vi "Main_TwoLoopsV3.vi"() -> ()   [LabVIEW 2022 SP3]
uses:
  SubVIs/ENUMs/StateENUM.ctl
  <vilib>/Instr/_visa.llb/VISA Configure Serial Port (Instr).vi
  <vilib>/ptbypt/NI_PtbyPt.lvlib
panel:
  in  "Enable PID":bool
  in  "Delay (sec)":dbl=5.0
  in  "Target Pressure":dbl=50.0
  out "Systole":dbl
  out "Diastole":dbl
  out "MAP":dbl
  out "Waveform Chart":dbl(graph)
  in  "Check Center":bool
  out "Step":i32
  in  "Increase Step":bool
  in  "Decrease Step":bool
  out "Center":i32
  out "LoopCount":i32
  in  "Jitter Up":bool
  in  "Jitter Down":bool
  out "Command Buffer":string
  in  "stop":bool
  out "Current Time":timestamp format="%<%I:%M:%S %p | %m/%d/%y>T"
  in  "VISA resource name":refnum<visa-resource-name>="COM9"
  in  "Up Button":bool
  in  "Down Button":bool
  # "Manual\nAdjustment"
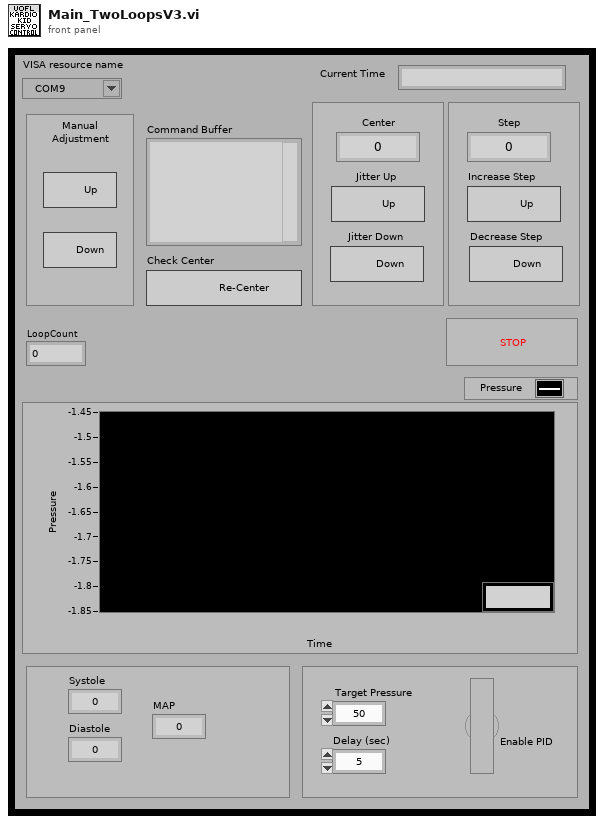
[diagram p1: front panel]
types:
  T1 = typedef "StateENUM.ctl" = enum16{"Init", "Idle", "MoveUp", "MoveDown", "JitterUp", "JitterDown", "IncreaseStep", "DecreaseStep", "CheckCenter", "ReadSerial", "ScanData", "Shutdown"}
  T2 = cluster{"Time Stamp":timestamp, "Delay":dbl, "PIDEnabled?":bool, "Target Pressure":dbl, "MAP":dbl}
  T3 = cluster{"State":T1, "Stop":bool, "error out":errorcluster}
  T4 = typedef "MoveCommands.ctl" = cluster{"MoveUp":string, "MoveDown":string, "JitterUp":string, "JitterDown":string, "IncStep":string, "DecStep":string, "ChkCenter":string}
  T5 = cluster{"VISA resource name out":refnum<visa-resource-name>, "error out":errorcluster, "State":T1, "Stop":bool, "Buffer":string, "Center":i32, "Step":i32, "SerialIncoming?":bool, "MoveCommands":T4}
  T6 = cluster{"Command Buffer":refnum<vi>, "Jitter Up":refnum<vi>, "Jitter Down":refnum<vi>, "Increase Step":refnum<vi>, "Decrease Step":refnum<vi>}
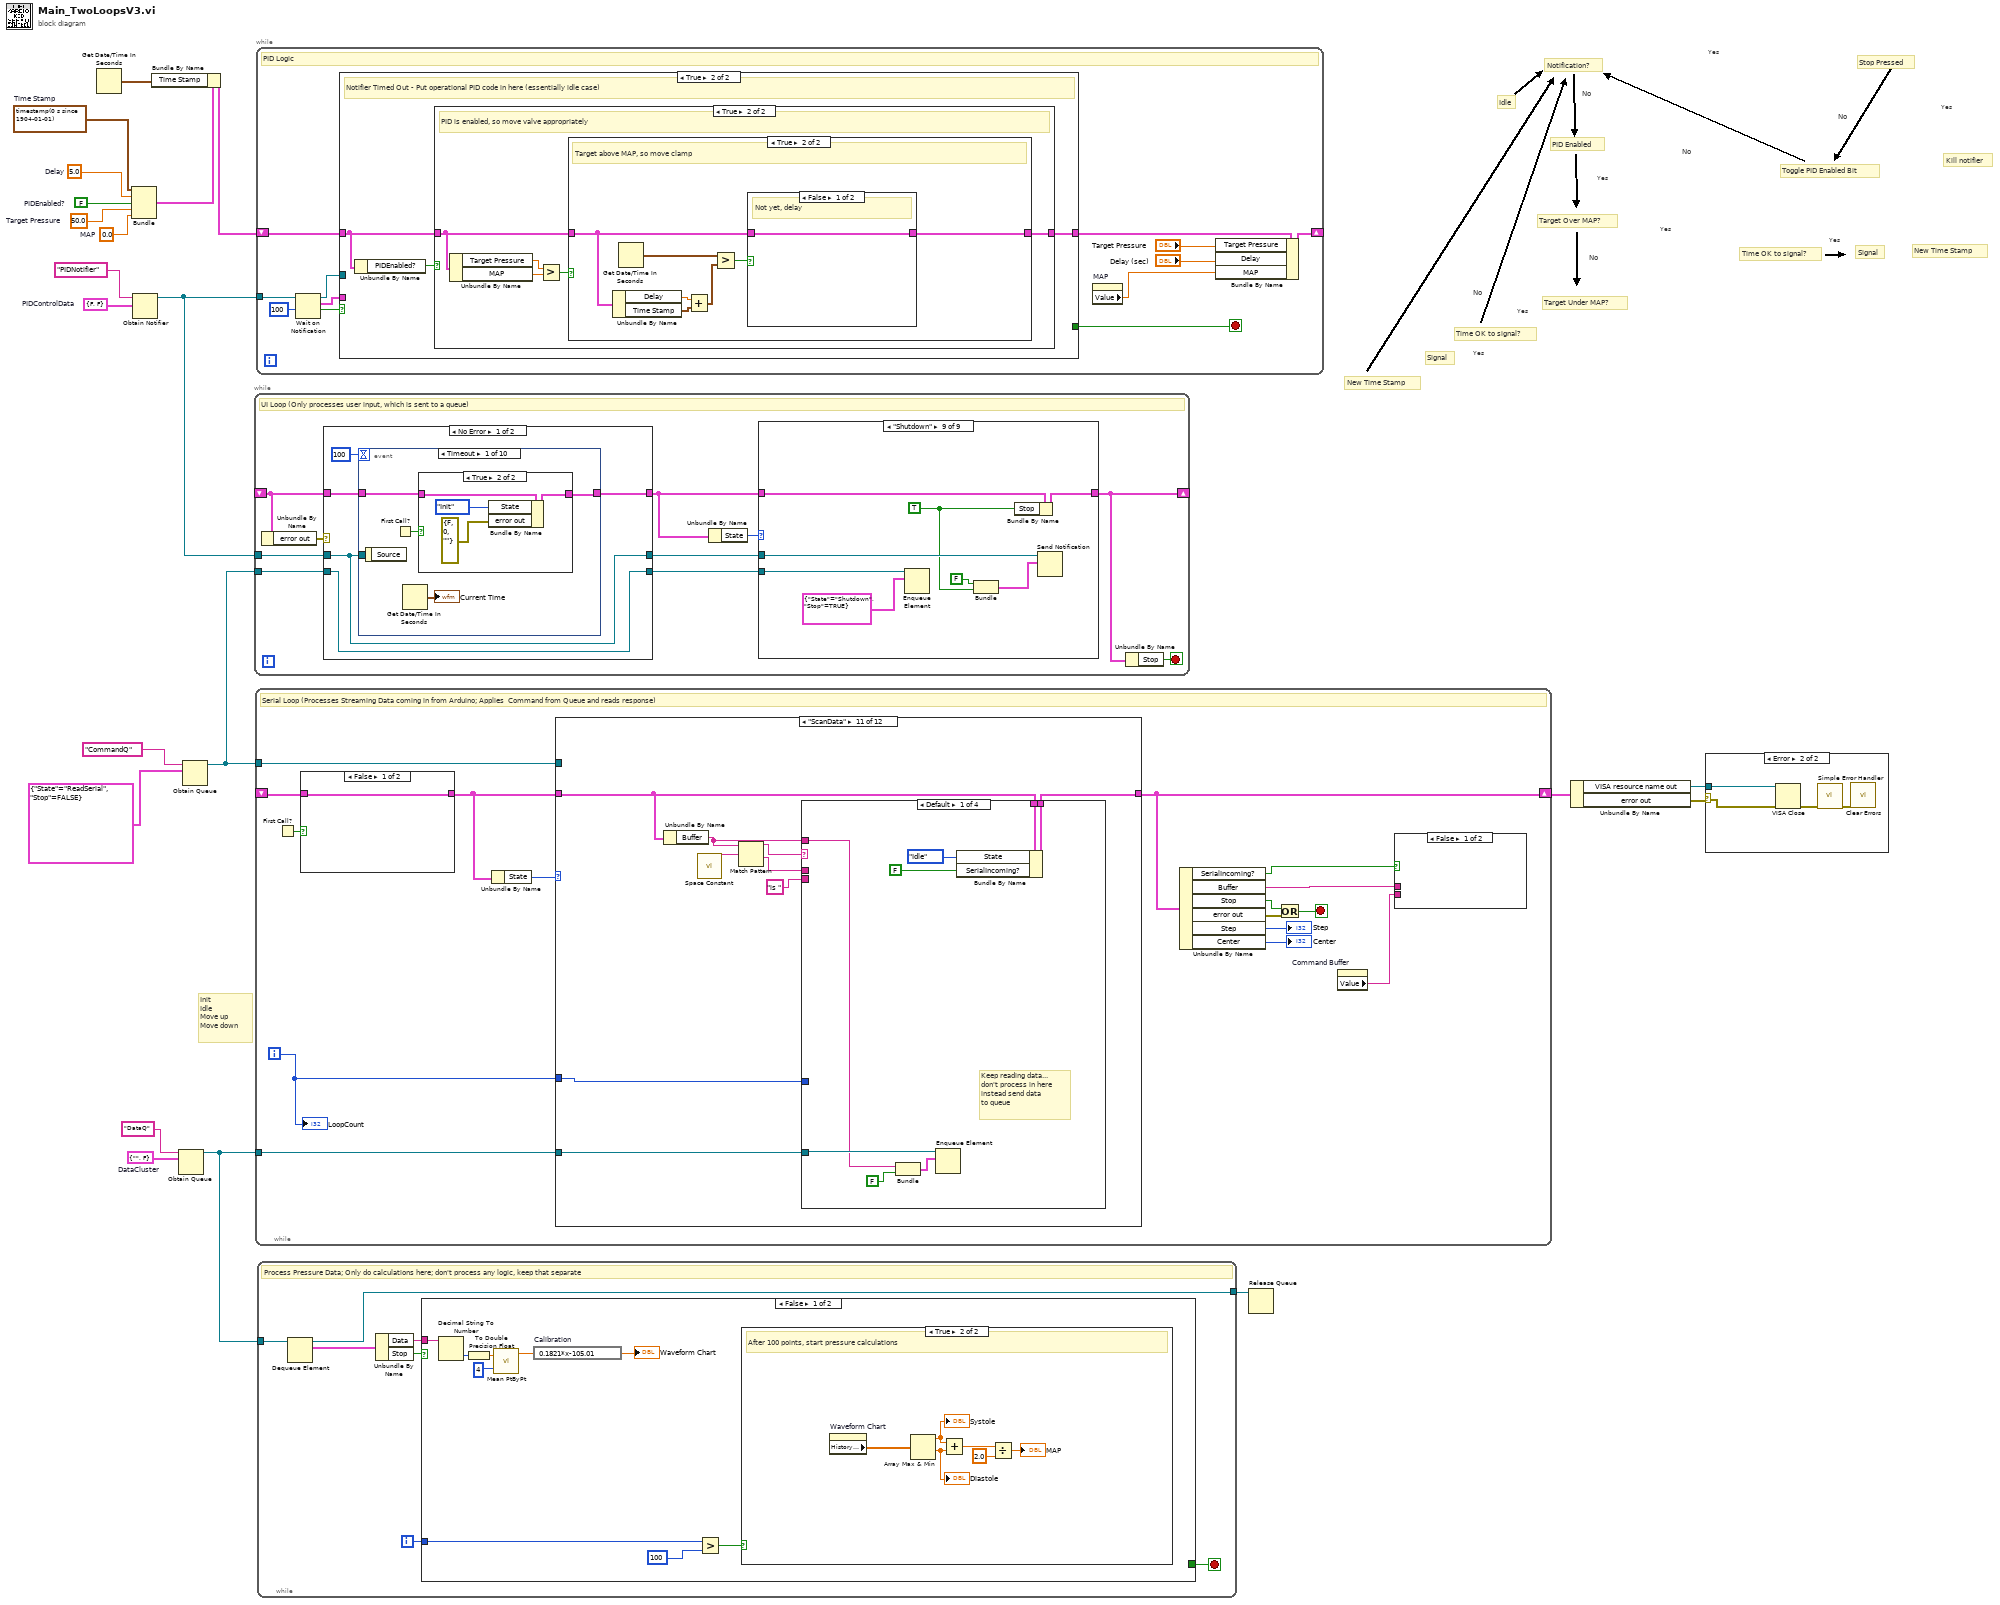
[diagram p0: block diagram]
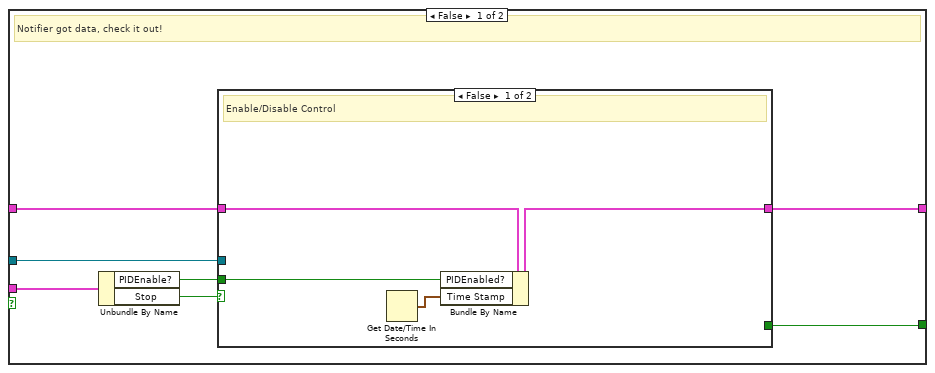
[diagram p2: hidden frame]
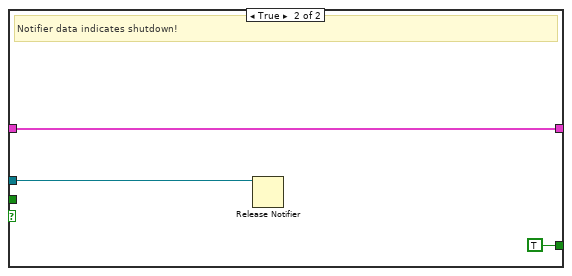
[diagram p3: hidden frame]
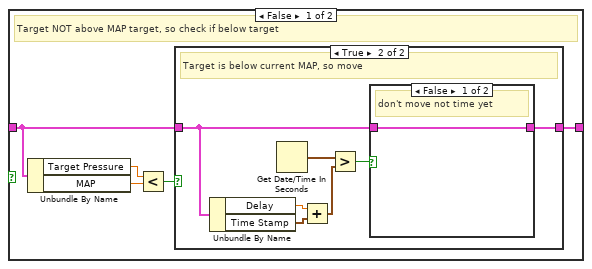
[diagram p5: hidden frame]
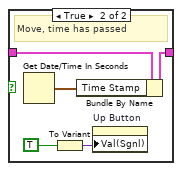
[diagram p7: hidden frame]
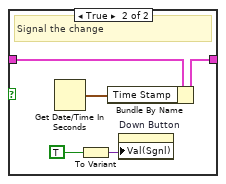
[diagram p8: hidden frame]
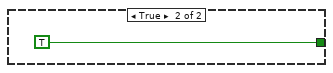
[diagram p10: hidden frame]
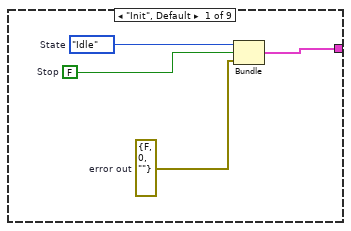
[diagram p11: hidden frame]
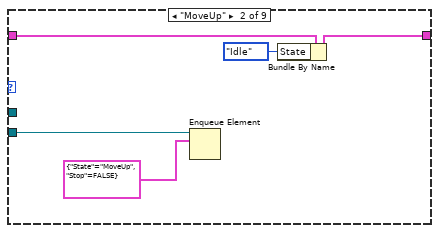
[diagram p12: hidden frame]
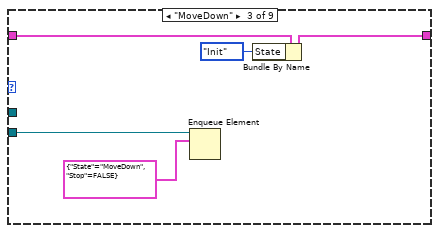
[diagram p13: hidden frame]
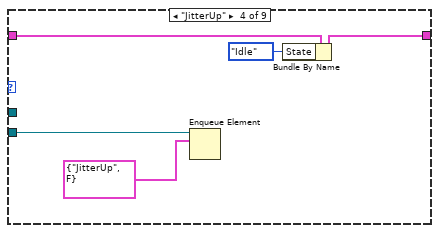
[diagram p14: hidden frame]
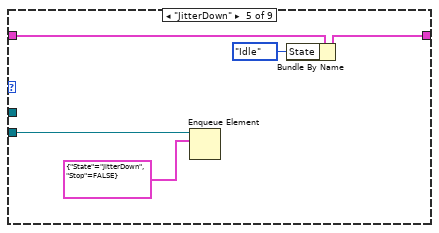
[diagram p15: hidden frame]
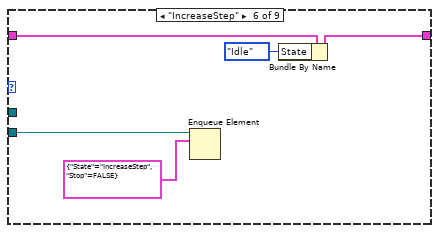
[diagram p16: hidden frame]
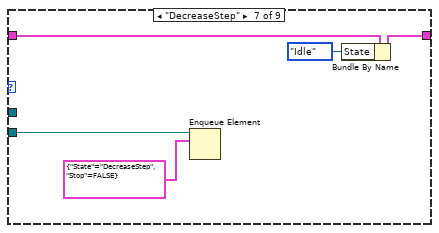
[diagram p17: hidden frame]
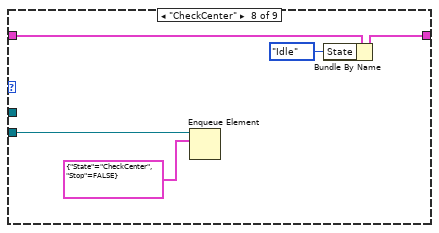
[diagram p18: hidden frame]
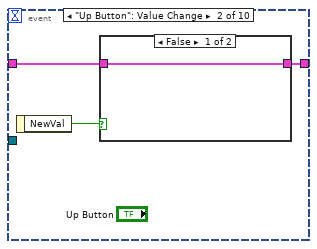
[diagram p20: hidden frame]
diagram:
  w2 = 0.0  # MAP
  w5 = timestamp(0 s since 1904-01-01)  # Time Stamp
  w6 = 5.0  # Delay
  w8 = 50.0  # Target Pressure
  w9 = FALSE  # PIDEnabled?
  w10 = cluster{"PIDEnable?":bool, "Stop":bool} {"PIDEnable?"=FALSE, "Stop"=FALSE}  # PIDControlData
  w14 = cluster{"Data":string, "Stop":bool} {"Data"="", "Stop"=FALSE}  # DataCluster
  # "No"
  # "Yes"
  # "New Time Stamp"
  # "Yes"
  # "Target Under MAP?"
  # "Time OK to signal?"
  # "Signal"
  # "No"
  # "Yes"
  # "New Time Stamp"
  # "Yes"
  # "Target Over MAP?"
  # "No"
  # "Yes"
  # "Time OK to signal?"
  # "Toggle PID Enabled Bit"
  # "No"
  # "Kill notifier"
  # "Yes"
  # "Stop Pressed"
  # "Notification?"
  # "Yes"
  # "Signal"
  # "No"
  # "Idle"
  # "PID Enabled"
  # "Init\nIdle\nMove up\nMove down"
  n1 = Get Date/Time In Seconds() -> (seconds since 1Jan1904=w3:timestamp)
  n2 = Bundle("Time Stamp"=w5, "Delay"=w6, "PIDEnabled?"=w9, "Target Pressure"=w8, "MAP"=w2) -> (w7:T2)  [unwired: 1 in]
  n3 = Obtain Notifier(name (unnamed)="PIDNotifier", notification data type=w10) -> (notifier out=w1:refnum<notifier>)  [unwired: 2 in, 2 out]
  n4 = Bundle By Name(cluster=w7, "Time Stamp"=w3) -> (w4:T2)
  n5 = Obtain Queue(name (unnamed)="DataQ", element data type=w14) -> (queue out=w13:refnum<queue>)  [unwired: 3 in, 2 out]
  n6 = Obtain Queue(name (unnamed)="CommandQ", element data type=cluster{"State":T1, "Stop":bool} {"State"=enum."ReadSerial", "Stop"=FALSE}) -> (queue out=w16:refnum<queue>)  [unwired: 3 in, 2 out]
  n7 = while {
    shift-right: [w30] -> _
    shift-left: _ -> [w28]
    tunnel: w16 -> [w26]
    tunnel: w1 -> [w23]
    stop <- w24 stop-if-true
    # "UI Loop (Only processes user input, which is sent to a queue)"
    n8 = Unbundle By Name(w28) -> ("error out"=w27:errorcluster)
    n9 = case shown="No Error" w27 {
      tunnel: w28 -> [w81 w161]
      tunnel: [w82 w157] -> w31
      tunnel: w26 -> [w80 w155]
      tunnel: [w80 w155] -> w25
      tunnel: w23 -> [w79 w154]
      tunnel: [w79 w154] -> w22
      frame No Error {
        n10 = event shown="[0] Timeout" {
          selector: _ -> [_ _ _ _ _ _ _ _ _ _]
          dyn-events: _ -> [_ _ _ _ _ _ _ _ _ _]
          timeout: 100 -> [_ _ _ _ _ _ _ _ _ _]
          tunnel: w81 -> [w85 w95 w104 w106 w114 w121 w128 w135 w142 w148]
          tunnel: [w84 w93 w104 w105 w112 w119 w126 w133 w140 w147] -> w82
          tunnel: w79 -> [_ _ w103 _ _ _ _ _ _ _]
          event Timeout {
            n11 = event-data() -> ()  [unwired: 1 in, 1 out]
            n12 = First Call?() -> (First Call?: T/F=w86:bool)
            n13 = Get Date/Time In Seconds() -> (seconds since 1Jan1904=→"Current Time":timestamp)
            n14 = case shown="True" w86 {
              tunnel: [w88 w91] -> w84
              tunnel: w85 -> [w88 w92]
              frame False {
              }
              frame True {
                n15 = Bundle By Name(cluster=w92, "State"=StateENUM."Init", "error out"=errorcluster {"status"=FALSE, "code"=0, "source"=""}) -> (w91:T3)
              }
            }
          }
          event "Up Button": Value Change {
            n16 = event-data() -> ("NewVal"=w94:bool)  [unwired: 1 in]
            n17 = case shown="False" w94 {
              tunnel: w95 -> [w96 w99]
              tunnel: [w96 w98] -> w93
              frame False {
              }
              frame True {
                n18 = Bundle By Name(cluster=w99, "State"=StateENUM."MoveUp") -> (w98:T3)
              }
            }
          }
          event "Enable PID": Value Change {
            n19 = event-data() -> ("NewVal"=w102:bool)  [unwired: 1 in]
            n20 = Bundle("NewVal"=w102, FALSE) -> (w100:cluster{"NewVal":bool, bool})  [unwired: 1 in]
            n21 = Send Notification(notification=w100, notifier=w103) -> ()  [unwired: 1 in, 2 out]
          }
          event "Down Button": Value Change {
            n22 = event-data() -> ("NewVal"=w107:bool)  [unwired: 1 in]
            n23 = case shown="True" w107 {
              tunnel: w106 -> [w108 w111]
              tunnel: [w108 w110] -> w105
              frame False {
              }
              frame True {
                n24 = Bundle By Name(cluster=w111, "State"=StateENUM."MoveDown") -> (w110:T3)
              }
            }
          }
          event "Jitter Up": Value Change {
            n25 = event-data() -> ("NewVal"=w113:bool)  [unwired: 1 in]
            n26 = case shown="True" w113 {
              tunnel: w114 -> [w115 w118]
              tunnel: [w115 w117] -> w112
              frame False {
              }
              frame True {
                n27 = Bundle By Name(cluster=w118, "State"=StateENUM."JitterUp") -> (w117:T3)
              }
            }
          }
          event "Jitter Down": Value Change {
            n28 = event-data() -> ("NewVal"=w120:bool)  [unwired: 1 in]
            n29 = case shown="True" w120 {
              tunnel: w121 -> [w122 w125]
              tunnel: [w122 w124] -> w119
              frame False {
              }
              frame True {
                n30 = Bundle By Name(cluster=w125, "State"=StateENUM."JitterDown") -> (w124:T3)
              }
            }
          }
          event "Increase Step": Value Change {
            n31 = event-data() -> ("NewVal"=w127:bool)  [unwired: 1 in]
            n32 = case shown="True" w127 {
              tunnel: w128 -> [w129 w132]
              tunnel: [w129 w131] -> w126
              frame False {
              }
              frame True {
                n33 = Bundle By Name(cluster=w132, "State"=StateENUM."IncreaseStep") -> (w131:T3)
              }
            }
          }
          event "Decrease Step": Value Change {
            n34 = event-data() -> ("NewVal"=w134:bool)  [unwired: 1 in]
            n35 = case shown="True" w134 {
              tunnel: w135 -> [w136 w139]
              tunnel: [w136 w138] -> w133
              frame False {
              }
              frame True {
                n36 = Bundle By Name(cluster=w139, "State"=StateENUM."DecreaseStep") -> (w138:T3)
              }
            }
          }
          event "Check Center": Value Change {
            n37 = event-data() -> ("NewVal"=w141:bool)  [unwired: 1 in]
            n38 = case shown="True" w141 {
              tunnel: w142 -> [w143 w146]
              tunnel: [w143 w145] -> w140
              frame False {
              }
              frame True {
                n39 = Bundle By Name(cluster=w146, "State"=StateENUM."CheckCenter") -> (w145:T3)
              }
            }
          }
          event "stop": Value Change {
            n40 = event-data() -> ("NewVal"=w149:bool)  [unwired: 1 in]
            n41 = case shown="True" w149 {
              tunnel: w148 -> [w150 w153]
              tunnel: [w150 w152] -> w147
              frame False {
              }
              frame True {
                n42 = Bundle By Name(cluster=w153, "State"=StateENUM."Shutdown") -> (w152:T3)
              }
            }
          }
        }
      }
      frame Error {
        n43 = Unbundle By Name(w161) -> ("error out"=w160:errorcluster)
        n44 = call <vilib>:"Simple Error Handler.vi"("error in (no error)"=w160) -> ("code out"=w158:i32, "error out"=w159:errorcluster)  [unwired: 4 in, 3 out]
        n45 = call <vilib>:"Clear Errors.vi"("error in (no error)"=w159, "specific error code to clear (0: all)"=w158) -> ()  [unwired: 4 in, 2 out]
        n46 = Bundle By Name(cluster=w161, "State"=StateENUM."Shutdown") -> (w157:T3)
      }
    }
    n47 = Unbundle By Name(w31) -> ("State"=w29:T1)
    n48 = case shown="\"Shutdown\"" w29 {
      tunnel: w31 -> [_ w38 w43 w48 w53 w58 w63 w68 w76]
      tunnel: [w33 w37 w42 w47 w52 w57 w62 w67 w75] -> w30
      tunnel: w25 -> [_ w40 w45 w50 w55 w60 w65 w70 w78]
      tunnel: w22 -> [_ _ _ _ _ _ _ _ w74]
      frame "Init", Default {
        w32 = errorcluster {"status"=FALSE, "code"=0, "source"=""}  # error out
        w34 = FALSE  # Stop
        w35 = StateENUM."Idle"  # State
        n49 = Bundle("State"=w35, "Stop"=w34, "error out"=w32) -> (w33:T3)  [unwired: 1 in]
      }
      frame "MoveUp" {
        n50 = Enqueue Element(queue=w40, element=cluster{"State":T1, "Stop":bool} {"State"=enum."MoveUp", "Stop"=FALSE}) -> ()  [unwired: 2 in, 3 out]
        n51 = Bundle By Name(cluster=w38, "State"=StateENUM."Idle") -> (w37:T3)
      }
      frame "MoveDown" {
        n52 = Enqueue Element(queue=w45, element=cluster{"State":T1, "Stop":bool} {"State"=enum."MoveDown", "Stop"=FALSE}) -> ()  [unwired: 2 in, 3 out]
        n53 = Bundle By Name(cluster=w43, "State"=StateENUM."Init") -> (w42:T3)
      }
      frame "JitterUp" {
        n54 = Enqueue Element(queue=w50, element=cluster{"State":T1, "Stop":bool} {"State"=enum."JitterUp", "Stop"=FALSE}) -> ()  [unwired: 2 in, 3 out]
        n55 = Bundle By Name(cluster=w48, "State"=StateENUM."Idle") -> (w47:T3)
      }
      frame "JitterDown" {
        n56 = Enqueue Element(queue=w55, element=cluster{"State":T1, "Stop":bool} {"State"=enum."JitterDown", "Stop"=FALSE}) -> ()  [unwired: 2 in, 3 out]
        n57 = Bundle By Name(cluster=w53, "State"=StateENUM."Idle") -> (w52:T3)
      }
      frame "IncreaseStep" {
        n58 = Enqueue Element(queue=w60, element=cluster{"State":T1, "Stop":bool} {"State"=enum."IncreaseStep", "Stop"=FALSE}) -> ()  [unwired: 2 in, 3 out]
        n59 = Bundle By Name(cluster=w58, "State"=StateENUM."Idle") -> (w57:T3)
      }
      frame "DecreaseStep" {
        n60 = Enqueue Element(queue=w65, element=cluster{"State":T1, "Stop":bool} {"State"=enum."DecreaseStep", "Stop"=FALSE}) -> ()  [unwired: 2 in, 3 out]
        n61 = Bundle By Name(cluster=w63, "State"=StateENUM."Idle") -> (w62:T3)
      }
      frame "CheckCenter" {
        n62 = Enqueue Element(queue=w70, element=cluster{"State":T1, "Stop":bool} {"State"=enum."CheckCenter", "Stop"=FALSE}) -> ()  [unwired: 2 in, 3 out]
        n63 = Bundle By Name(cluster=w68, "State"=StateENUM."Idle") -> (w67:T3)
      }
      frame "Shutdown" {
        w73 = TRUE ("Stop")
        n64 = Enqueue Element(queue=w78, element=cluster{"State":T1, "Stop":bool} {"State"=enum."Shutdown", "Stop"=TRUE}) -> ()  [unwired: 2 in, 3 out]
        n65 = Bundle("Stop"=FALSE, "Stop"=w73) -> (w71:cluster{"Stop":bool, "Stop":bool})  [unwired: 1 in]
        n66 = Bundle By Name(cluster=w76, "Stop"=w73) -> (w75:T3)
        n67 = Send Notification(notification=w71, notifier=w74) -> ()  [unwired: 1 in, 2 out]
      }
    }
    n68 = Unbundle By Name(w30) -> ("Stop"=w24:bool)
  }
  n69 = while {
    shift-right: [w176] -> w21
    shift-left: _ -> [w166]
    tunnel: w16 -> [w164]
    tunnel: w13 -> [w162]
    i -> [w163]
    stop <- w175 stop-if-true
    # "Serial Loop (Processes Streaming Data coming in from Arduino; Applies  Command from Queue and reads response)"
    n70 = First Call?() -> (First Call?: T/F=w167:bool)
    n71 = case shown="False" w167 {
      tunnel: [w178 w181] -> w165
      tunnel: w166 -> [w178 w182]
      frame False {
      }
      frame True {
        n72 = Bundle By Name(cluster=w182, "State"=StateENUM."Init", "error out"=errorcluster {"status"=FALSE, "code"=0, "source"=""}) -> (w181:T5)
      }
    }
    n73 = Unbundle By Name(w165) -> ("State"=w177:T1)
    n74 = case shown="\"ScanData\"" w177 {
      tunnel: [w206 w211 w234 w241 w249 w258 w265 w272 w279 w294 w314 w353] -> w176
      tunnel: w165 -> [_ w212 w235 w242 w251 w260 w267 w274 w281 w295 w315 w355]
      tunnel: w164 -> [_ w210 _ _ _ _ _ _ _ _ _ w348]
      tunnel: w163 -> [_ _ _ _ _ _ _ _ _ _ w308 _]
      tunnel: w162 -> [_ _ _ _ _ _ _ _ _ _ w307 _]
      frame "Init", Default {
        w194 = FALSE  # SerialIncoming?
        w196 = 50  # Step
        w197 = 1500  # Center
        w199 = ""  # Buffer
        w204 = FALSE  # Stop
        w205 = StateENUM."Idle"  # State
        n75 = property on="Command Buffer" class="Str"("Value"="") -> ()  [unwired: 2 in, 2 out]
        n76 = call-poly "VISA Configure Serial Port"("VISA resource name"="VISA resource name") -> ("VISA resource name out"=w202:refnum<visa-resource-name>, "error out"=w201:errorcluster)  [unwired: 13 in]
        n77 = VISA Flush I/O Buffer(VISA resource name=w202, error in (no error)=w201) -> (VISA resource name out=w195:refnum<visa-resource-name>, error out=w200:errorcluster)  [unwired: 1 in]
        n78 = control-ref of="Jitter Up"() -> (w189:refnum<vi>)
        n79 = control-ref of="Jitter Down"() -> (w190:refnum<vi>)
        n80 = control-ref of="Increase Step"() -> (w191:refnum<vi>)
        n81 = control-ref of="Decrease Step"() -> (w192:refnum<vi>)
        n82 = control-ref of="Command Buffer"() -> (w188:refnum<vi>)
        n83 = Bundle("Command Buffer"=w188, "Jitter Up"=w189, "Jitter Down"=w190, "Increase Step"=w191, "Decrease Step"=w192) -> (w187:T6)  [unwired: 1 in]
        n84 = call "MoveCommands (SubVI).vi"() -> ("MoveCommands"=w193:T4)  [unwired: 11 in]
        n85 = call "InitPostions (SubVI).vi"("ControlCluster"=w187) -> ()  [unwired: 11 in]
        n86 = Wait (ms)(milliseconds to wait=u32 5) -> ()  [unwired: 1 out]
        n87 = Bundle("VISA resource name out"=w195, "error out"=w200, "State"=w205, "Stop"=w204, "Buffer"=w199, "Center"=w197, "Step"=w196, "SerialIncoming?"=w194, "MoveCommands"=w193) -> (w206:T5)  [unwired: 1 in]
      }
      frame "Idle" {
        n88 = Dequeue Element(queue=w210, timeout in ms (-1)=10) -> (element=w208:cluster{"State":T1, "Stop":bool}, timed out?=w209:bool)  [unwired: 1 in, 2 out]
        n89 = case shown="True" w209 {
          tunnel: w212 -> [w216 w228]
          tunnel: [w215 w226] -> w211
          tunnel: w208 -> [w214 _]
          frame False {
            n90 = Unbundle By Name(w214) -> ("State"=w213:T1)
            n91 = Bundle By Name(cluster=w216, "State"=w213) -> (w215:T5)
          }
          frame True {
            w220 = StateENUM."ReadSerial"  # State
            n92 = Unbundle By Name(w228) -> ("State"=w219:T1, "VISA resource name out"=w225:refnum<visa-resource-name>, "error out"=w224:errorcluster)
            n93 = Wait (ms)(milliseconds to wait=u32 5) -> ()  [unwired: 1 out]
            n94 = property class="Instr"(reference=w225, error in=w224) -> (error out=w223:errorcluster, "Serial Settings:Number of Bytes at Serial Port"=w221:u32)  [unwired: 1 out]
            n95 = Greater Than 0?(x=w221) -> (x > 0?=w218:bool)
            n96 = Select(t=w220, s=w218, f=w219) -> (s? t:f=w222:T1)
            n97 = Bundle By Name(cluster=w228, "State"=w222, "error out"=w223, "SerialIncoming?"=FALSE) -> (w226:T5)
          }
        }
      }
      frame "MoveUp" {
        # "48 ASCII"
        n98 = Unbundle By Name(w235) -> ("VISA resource name out"=w230:refnum<visa-resource-name>, "MoveCommands.MoveUp"=w229:string, "error out"=w231:errorcluster)
        n99 = VISA Write(VISA resource name=w230, write buffer=w229, error in (no error)=w231) -> (error out=w232:errorcluster)  [unwired: 2 out]
        n100 = Bundle By Name(cluster=w235, "State"=StateENUM."ReadSerial", "error out"=w232) -> (w234:T5)
      }
      frame "MoveDown" {
        # "49 ASCII"
        n101 = Unbundle By Name(w242) -> ("VISA resource name out"=w237:refnum<visa-resource-name>, "MoveCommands.MoveDown"=w236:string, "error out"=w238:errorcluster)
        n102 = VISA Write(VISA resource name=w237, write buffer=w236, error in (no error)=w238) -> (error out=w239:errorcluster)  [unwired: 2 out]
        n103 = Bundle By Name(cluster=w242, "State"=StateENUM."ReadSerial", "error out"=w239) -> (w241:T5)
      }
      frame "JitterUp" {
        n104 = Unbundle By Name(w251) -> ("Center"=w246:i32, "VISA resource name out"=w250:refnum<visa-resource-name>, "MoveCommands.JitterUp"=w243:string, "error out"=w244:errorcluster)
        n105 = Increment(x=w246) -> (x+1=w245:i32)
        n106 = VISA Write(VISA resource name=w250, write buffer=w243, error in (no error)=w244) -> (error out=w247:errorcluster)  [unwired: 2 out]
        n107 = Bundle By Name(cluster=w251, "State"=StateENUM."ReadSerial", "Center"=w245, "error out"=w247) -> (w249:T5)
      }
      frame "JitterDown" {
        n108 = Unbundle By Name(w260) -> ("Center"=w255:i32, "VISA resource name out"=w259:refnum<visa-resource-name>, "MoveCommands.JitterDown"=w252:string, "error out"=w253:errorcluster)
        n109 = Decrement(x=w255) -> (x-1=w254:i32)
        n110 = VISA Write(VISA resource name=w259, write buffer=w252, error in (no error)=w253) -> (error out=w256:errorcluster)  [unwired: 2 out]
        n111 = Bundle By Name(cluster=w260, "State"=StateENUM."ReadSerial", "Center"=w254, "error out"=w256) -> (w258:T5)
      }
      frame "IncreaseStep" {
        n112 = Unbundle By Name(w267) -> ("VISA resource name out"=w266:refnum<visa-resource-name>, "MoveCommands.IncStep"=w261:string, "error out"=w262:errorcluster)
        n113 = VISA Write(VISA resource name=w266, write buffer=w261, error in (no error)=w262) -> (error out=w263:errorcluster)  [unwired: 2 out]
        n114 = Bundle By Name(cluster=w267, "State"=StateENUM."ReadSerial", "error out"=w263) -> (w265:T5)
      }
      frame "DecreaseStep" {
        n115 = Unbundle By Name(w274) -> ("VISA resource name out"=w273:refnum<visa-resource-name>, "MoveCommands.DecStep"=w269:string, "error out"=w268:errorcluster)
        n116 = VISA Write(VISA resource name=w273, write buffer=w269, error in (no error)=w268) -> (error out=w270:errorcluster)  [unwired: 2 out]
        n117 = Bundle By Name(cluster=w274, "State"=StateENUM."ReadSerial", "error out"=w270) -> (w272:T5)
      }
      frame "CheckCenter" {
        n118 = Unbundle By Name(w281) -> ("VISA resource name out"=w280:refnum<visa-resource-name>, "MoveCommands.ChkCenter"=w275:string, "error out"=w276:errorcluster)
        n119 = VISA Write(VISA resource name=w280, write buffer=w275, error in (no error)=w276) -> (error out=w277:errorcluster)  [unwired: 2 out]
        n120 = Bundle By Name(cluster=w281, "State"=StateENUM."ReadSerial", "error out"=w277) -> (w279:T5)
      }
      frame "ReadSerial" {
        n121 = Unbundle By Name(w295) -> ("VISA resource name out"=w290:refnum<visa-resource-name>, "error out"=w285:errorcluster, "Buffer"=w284:string)
        n122 = Wait (ms)(milliseconds to wait=u32 5) -> ()  [unwired: 1 out]
        n123 = property class="Instr"(reference=w290, error in=w285) -> (reference out=w287:refnum<visa-resource-name>, error out=w286:errorcluster, "Serial Settings:Number of Bytes at Serial Port"=w288:u32)
        n124 = Greater Than 0?(x=w288) -> (x > 0?=w289:bool)
        n125 = case shown="True" w289 {
          tunnel: [w298 w306] -> w292
          tunnel: [w299 w305] -> w291
          tunnel: w286 -> [w299 w304]
          tunnel: w287 -> [_ w303]
          tunnel: w288 -> [_ w302]
          tunnel: w284 -> [w298 _]
          tunnel: [StateENUM."Idle" ("State") StateENUM."ScanData" ("State")] -> w283
          tunnel: [FALSE FALSE] -> w282
          frame False {
          }
          frame True {
            n126 = VISA Read(VISA resource name=w303, byte count=w302, error in (no error)=w304) -> (read buffer=w306:string, error out=w305:errorcluster)  [unwired: 2 out]
          }
        }
        n127 = Bundle By Name(cluster=w295, "State"=w283, "SerialIncoming?"=w282, "Buffer"=w292, "error out"=w291) -> (w294:T5)
      }
      frame "ScanData" {
        n128 = Unbundle By Name(w315) -> ("Buffer"=w309:string)
        n129 = call <vilib>:"Space Constant.vi"() -> ("String"=w311:string)
        n130 = Match Pattern(string=w309, regular expression=w311) -> (before substring=w310:string, after substring=w312:string)  [unwired: 1 in, 2 out]
        n131 = case shown="Default" w310 {
          tunnel: "is " -> [_ _ w337 w347]
          tunnel: w312 -> [_ _ w336 w346]
          tunnel: w315 -> [w323 w327 w332 w342]
          tunnel: [w322 w326 w330 w340] -> w314
          tunnel: w309 -> [w318 _ _ _]
          tunnel: w308 -> [_ _ _ _]
          tunnel: w307 -> [w319 _ _ _]
          frame Default {
            # "Keep reading data...\ndon't process in here\ninstead send data\nto queue"
            n132 = Bundle("Buffer"=w318, FALSE) -> (w316:cluster{"Buffer":string, bool})  [unwired: 1 in]
            n133 = Enqueue Element(queue=w319, element=w316) -> ()  [unwired: 2 in, 3 out]
            n134 = Bundle By Name(cluster=w323, "State"=StateENUM."Idle", "SerialIncoming?"=FALSE) -> (w322:T5)
          }
          frame "Moving" {
            n135 = Bundle By Name(cluster=w327, "State"=StateENUM."Idle", "SerialIncoming?"=TRUE) -> (w326:T5)
          }
          frame "Center", "Stop" {
            n136 = Match Pattern(string=w336, regular expression=w337) -> (after substring=w334:string)  [unwired: 1 in, 3 out]
            n137 = Match Pattern(string=w334, regular expression="\r\n") -> (before substring=w333:string)  [unwired: 1 in, 3 out]
            n138 = Decimal String To Number(string=w333) -> (number=w331:i32)  [unwired: 2 in, 1 out]
            n139 = Bundle By Name(cluster=w332, "SerialIncoming?"=TRUE, "State"=StateENUM."Idle", "Center"=w331) -> (w330:T5)
          }
          frame "Step" {
            n140 = Match Pattern(string=w346, regular expression=w347) -> (after substring=w344:string)  [unwired: 1 in, 3 out]
            n141 = Match Pattern(string=w344, regular expression="\r\n") -> (before substring=w343:string)  [unwired: 1 in, 3 out]
            n142 = Decimal String To Number(string=w343) -> (number=w341:i32)  [unwired: 2 in, 1 out]
            n143 = Bundle By Name(cluster=w342, "SerialIncoming?"=TRUE, "State"=StateENUM."Idle", "Step"=w341) -> (w340:T5)
          }
        }
      }
      frame "Shutdown" {
        n144 = Release Queue(queue=w348) -> ()  [unwired: 2 in, 3 out]
        n145 = Unbundle By Name(w355) -> ("VISA resource name out"=w354:refnum<visa-resource-name>, "error out"=w349:errorcluster)
        n146 = VISA Close(VISA resource name=w354, error in (no error)=w349) -> (error out=w350:errorcluster)
        n147 = Bundle By Name(cluster=w355, "Stop"=TRUE, "State"=StateENUM."Shutdown", "error out"=w350) -> (w353:T5)
      }
    }
    n148 = Unbundle By Name(w176) -> ("SerialIncoming?"=w168:bool, "Buffer"=w172:string, "Stop"=w174:bool, "error out"=w173:errorcluster, "Step"=→"Step":i32, "Center"=→"Center":i32)
    n149 = Or(x=w174, y=w173) -> (x .or. y?=w175:bool)
    n150 = property on="Command Buffer" class="Str"() -> ("Value"=w171:string)  [unwired: 2 in, 2 out]
    n151 = case shown="False" w168 {
      tunnel: w172 -> [_ w185]
      tunnel: w171 -> [_ w184]
      frame False {
      }
      frame True {
        n152 = Concatenate Strings(w185, w184) -> (→"Command Buffer":string)
      }
    }
    "LoopCount" <- w163
  }
  n153 = while {
    tunnel: w1 -> [w367]
    shift-right: [w360] -> _
    shift-left: w4 -> [w362]
    stop <- w364 stop-if-true
    # "PID Logic"
    n154 = Wait on Notification(notifier=w367, timeout in ms (-1)=100) -> (notifier out=w356:refnum<notifier>, notification=w363:cluster{"PIDEnable?":bool, "Stop":bool}, timed out?=w365:bool)  [unwired: 2 in, 1 out]
    n155 = case shown="True" w365 {
      tunnel: [w369 _] -> w364
      tunnel: w363 -> [w374 _]
      tunnel: w362 -> [w372 w383]
      tunnel: [w371 w382] -> w361
      tunnel: w356 -> [w368 _]
      frame False {
        # "Notifier got data, check it out!"
        n156 = Unbundle By Name(w374) -> ("PIDEnable?"=w370:bool, "Stop"=w373:bool)
        n157 = case shown="False" w373 {
          tunnel: w372 -> [w378 w381]
          tunnel: [w376 w381] -> w371
          tunnel: w370 -> [w377 _]
          tunnel: [_ TRUE] -> w369
          tunnel: w368 -> [_ w379]
          frame False {
            # "Enable/Disable Control"
            n158 = Get Date/Time In Seconds() -> (seconds since 1Jan1904=w375:timestamp)
            n159 = Bundle By Name(cluster=w378, "PIDEnabled?"=w377, "Time Stamp"=w375) -> (w376:T2)
          }
          frame True {
            # "Notifier data indicates shutdown!"
            n160 = Release Notifier(notifier=w379) -> ()  [unwired: 2 in, 3 out]
          }
        }
      }
      frame True {
        # "Notifier Timed Out - Put operational PID code in here (essentially idle case)"
        n161 = Unbundle By Name(w383) -> ("PIDEnabled?"=w384:bool)
        n162 = case shown="True" w384 {
          tunnel: w383 -> [w385 w387]
          tunnel: [w385 w386] -> w382
          frame False {
            # "PID is not enabled, so don't do anything...."
          }
          frame True {
            # "PID is enabled, so move valve appropriately"
            n163 = Unbundle By Name(w387) -> ("Target Pressure"=w389:dbl, "MAP"=w388:dbl)
            n164 = Greater?(x=w389, y=w388) -> (0:w390:bool)
            n165 = case shown="True" w390 {
              tunnel: w387 -> [w392 w415]
              tunnel: [w395 w416] -> w386
              frame False {
                # "Target NOT above MAP target, so check if below target"
                n166 = Unbundle By Name(w392) -> ("Target Pressure"=w393:dbl, "MAP"=w394:dbl)
                n167 = Less?(x=w393, y=w394) -> (x < y?=w391:bool)
                n168 = case shown="True" w391 {
                  tunnel: [w396 w403] -> w395
                  tunnel: w392 -> [w396 w397]
                  frame False {
                  }
                  frame True {
                    # "Target is below current MAP, so move"
                    n169 = Unbundle By Name(w397) -> ("Delay"=w402:dbl, "Time Stamp"=w401:timestamp)
                    n170 = Get Date/Time In Seconds() -> (seconds since 1Jan1904=w400:timestamp)
                    n171 = Add(x=w402, y=w401) -> (x+y=w399:timestamp)
                    n172 = Greater?(x=w400, y=w399) -> (0:w398:bool)
                    n173 = case shown="False" w398 {
                      tunnel: [w404 w409] -> w403
                      tunnel: w397 -> [w404 w408]
                      frame False {
                        # "don't move not time yet"
                      }
                      frame True {
                        # "Move, time has passed"
                        n174 = Get Date/Time In Seconds() -> (seconds since 1Jan1904=w406:timestamp)
                        n175 = To Variant(anything=TRUE) -> (Variant=w405:variant)
                        n176 = Bundle By Name(cluster=w408, "Time Stamp"=w406) -> (w409:T2)
                        n177 = property on="Up Button" class="Bool"("Val(Sgnl)"=w405) -> ()  [unwired: 2 in, 2 out]
                      }
                    }
                  }
                }
              }
              frame True {
                # "Target above MAP, so move clamp"
                n178 = Unbundle By Name(w415) -> ("Delay"=w414:dbl, "Time Stamp"=w413:timestamp)
                n179 = Get Date/Time In Seconds() -> (seconds since 1Jan1904=w412:timestamp)
                n180 = Add(x=w414, y=w413) -> (x+y=w411:timestamp)
                n181 = Greater?(x=w412, y=w411) -> (0:w410:bool)
                n182 = case shown="False" w410 {
                  tunnel: [w417 w422] -> w416
                  tunnel: w415 -> [w417 w421]
                  frame False {
                    # "Not yet, delay"
                  }
                  frame True {
                    # "Signal the change"
                    n183 = Get Date/Time In Seconds() -> (seconds since 1Jan1904=w418:timestamp)
                    n184 = To Variant(anything=TRUE) -> (Variant=w420:variant)
                    n185 = Bundle By Name(cluster=w421, "Time Stamp"=w418) -> (w422:T2)
                    n186 = property on="Down Button" class="Bool"("Val(Sgnl)"=w420) -> ()  [unwired: 2 in, 2 out]
                  }
                }
              }
            }
          }
        }
      }
    }
    n187 = property on="MAP" class="DigNum (strict)"() -> ("Value"=w357:dbl)  [unwired: 2 in, 2 out]
    n188 = Bundle By Name(cluster=w361, "Target Pressure"="Target Pressure", "Delay"="Delay (sec)", "MAP"=w357) -> (w360:T2)
  }
  n189 = while {
    tunnel: w13 -> [w429]
    tunnel: [w423] -> w12
    i -> [w424]
    stop <- w425 stop-if-true
    # "Process Pressure Data; Only do calculations here; don't process any logic, keep that separate"
    n190 = Dequeue Element(queue=w429) -> (queue out=w423:refnum<queue>, element=w427:cluster{"Data":string, "Stop":bool})  [unwired: 2 in, 2 out]
    n191 = Unbundle By Name(w427) -> ("Data"=w426:string, "Stop"=w428:bool)
    n192 = case shown="False" w428 {
      tunnel: w426 -> [w436 _]
      tunnel: [_ TRUE] -> w425
      tunnel: w424 -> [w433 _]
      frame False {
        n193 = Decimal String To Number(string=w436) -> (number=w437:i32)  [unwired: 2 in, 1 out]
        n194 = To Double Precision Float(number=w437) -> (double precision float=w435:dbl)
        n195 = call <vilib>:"Mean PtByPt.vi"("x"=w435, "sample length"=4) -> ("mean"=w431:dbl)  [unwired: 2 in, 1 out]
        n196 = expression code="0.1821*x-105.01" "Calibration"(w431) -> (→"Waveform Chart":dbl)
        n197 = Greater?(x=w433, y=100) -> (0:w434:bool)
        n198 = case shown="True" w434 {
          frame False {
          }
          frame True {
            # "After 100 points, start pressure calculations"
            n199 = property on="Waveform Chart" class="WFChart (strict)"() -> ("History Data"=w444:dbl[])  [unwired: 2 in, 2 out]
            n200 = Array Max & Min(array=w444) -> (max value=w440:dbl, min value=w441:dbl)  [unwired: 2 out]
            "Systole" <- w440
            "Diastole" <- w441
            n201 = Add(x=w440, y=w441) -> (x+y=w443:dbl)
            n202 = Divide(x=w443, y=2.0) -> (x/y=→"MAP":dbl)
          }
        }
      }
      frame True {
      }
    }
  }
  n203 = Release Queue(queue=w12) -> ()  [unwired: 2 in, 3 out]
  n204 = Unbundle By Name(w21) -> ("VISA resource name out"=w19:refnum<visa-resource-name>, "error out"=w20:errorcluster)
  n205 = case shown="Error" w20 {
    selector: w20 -> [_ w447]
    tunnel: w19 -> [_ w449]
    frame No Error {
    }
    frame Error {
      n206 = VISA Close(VISA resource name=w449, error in (no error)=w447) -> (error out=w446:errorcluster)
      n207 = call <vilib>:"Simple Error Handler.vi"("error in (no error)"=w446) -> ("error out"=w448:errorcluster)  [unwired: 4 in, 4 out]
      n208 = call <vilib>:"Clear Errors.vi"("error in (no error)"=w448) -> ()  [unwired: 5 in, 2 out]
    }
  }
